vi "Charts Modes.vi"() -> ()   [LabVIEW 2024]
panel:
  out "Sweep Chart":dbl(graph)
  out "Scope Chart":dbl(graph)
  out "Strip Chart":dbl(graph)
  out "Out":dbl[](array[numeric])
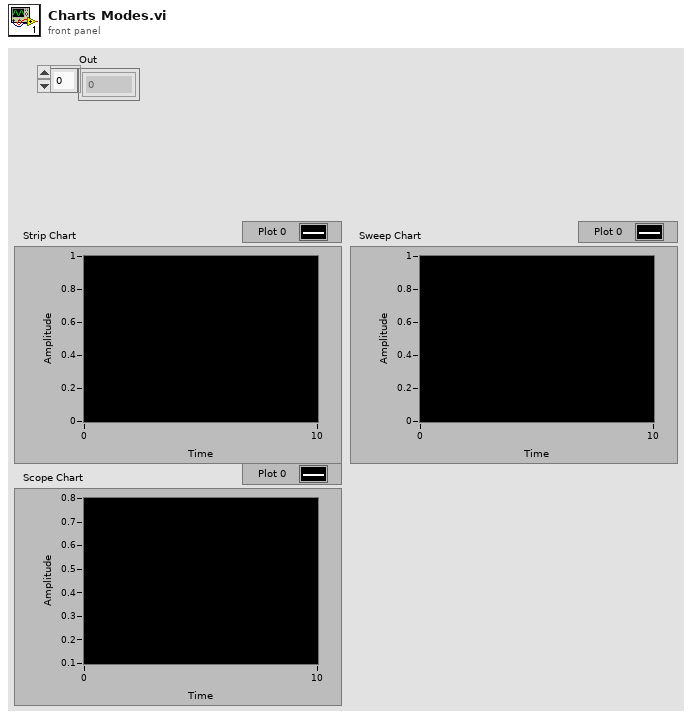
[diagram p1: front panel]
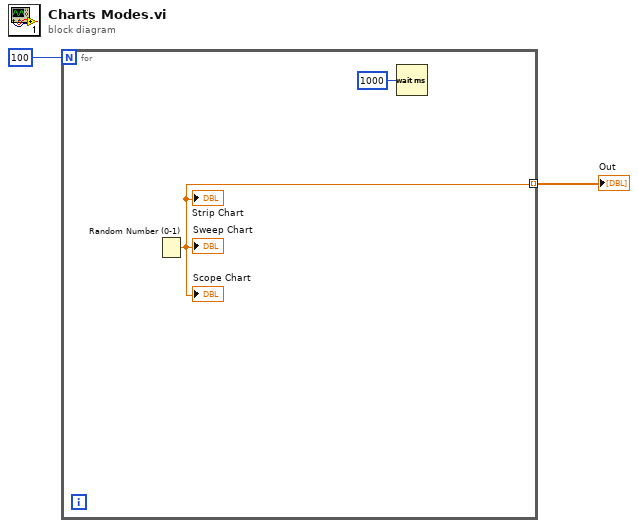
[diagram p0: block diagram]
diagram:
  n1 = for {
    N: 100 -> [_]
    tunnel: [w3] -> w1 mode=indexing
    n2 = Random Number (0-1)() -> (number: 0 to 1=w3:dbl)
    "Strip Chart" <- w3
    "Scope Chart" <- w3
    "Sweep Chart" <- w3
    n3 = Wait (ms)(milliseconds to wait=u32 1000) -> ()  [unwired: 1 out]
  }
  "Out" <- w1
